vi "Initialize-object.vi"(8 "error in (no error)":errorcluster, 10 "Settings":T1, 11 "Base path":path) -> (0 "error out":errorcluster, 3 "Errors out":T3)   [LabVIEW 2013, in "CameraVision.lvlib" / "CV-Errors.lvclass"]
uses:
  CV-Errors.lvclass
  Object-reference.ctl
  Settings.ctl
  Languages.ctl
  CV-Errors.lvclass/CV-Errors.ctl
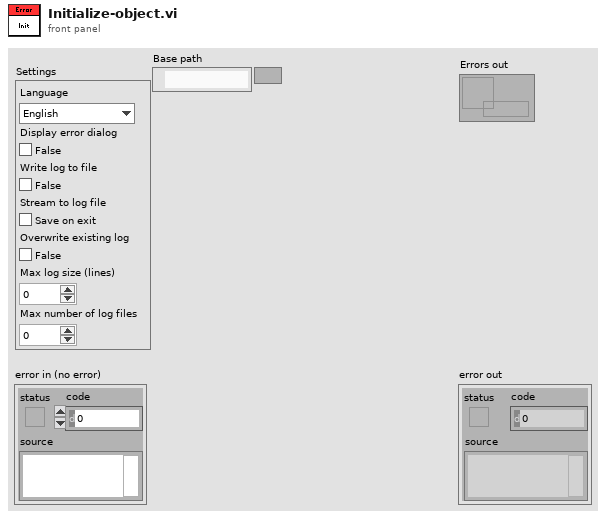
[diagram p1: front panel]
types:
  T1 = typedef "CameraVision.lvlib/CV-Errors.lvclass/Settings.ctl" = cluster{"Language":T2, "Display error dialog":bool, "Write log to file":bool, "Stream to log file":bool, "Overwrite existing log":bool, "Max log size":i32, "Max number of log files":i32}
  T2 = typedef "CameraVision.lvlib/CV-Errors.lvclass/Languages.ctl" = enum16{"English"}
  T3 = typedef "CameraVision.lvlib/CV-Errors.lvclass/Object-reference.ctl" = refnum<data-value>
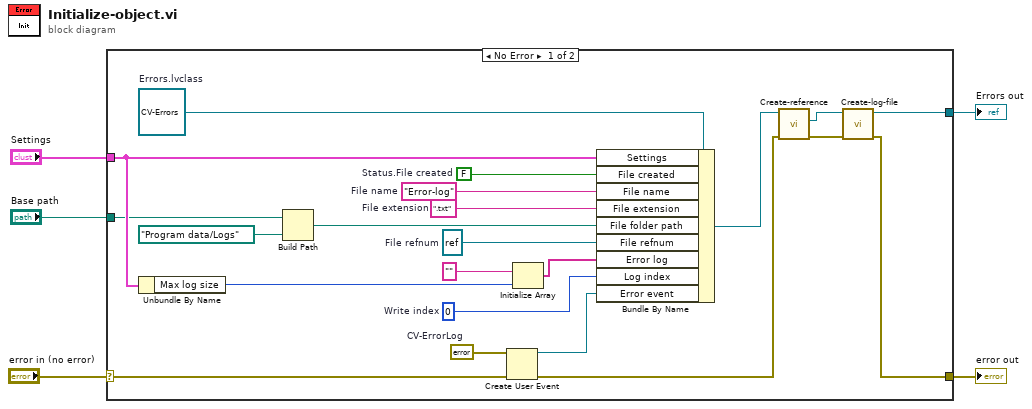
[diagram p0: block diagram]
diagram:
  n1 = case shown="No Error" "error in (no error)" {
    selector: "error in (no error)" -> [w9 w28]
    tunnel: [w17 w28] -> w4
    tunnel: [w16 _] -> w3
    tunnel: "Settings" -> [w13 _]
    tunnel: "Base path" -> [w7 _]
    frame No Error {
      w8 = errorcluster {"status"=FALSE, "code"=0, "source"=""}  # CV-ErrorLog
      w14 = FALSE  # Status.File created
      w15 = refnum<class "CV-Errors.lvclass"> refnum  # Errors.lvclass
      w21 = 0  # Write index
      w24 = refnum<file> refnum  # File refnum
      w26 = ".txt"  # File extension
      w27 = "Error-log"  # File name
      n2 = Unbundle By Name(w13) -> ("Max log size"=w12:i32)
      n3 = Build Path(base path=w7, name or relative path=path "Program data/Logs") -> (appended path=w25:path)
      n4 = Create User Event(user event datatype=w8, error in=w9) -> (user event=w10:refnum<user-event>, error out=w11:errorcluster)
      n5 = Initialize Array("", w12) -> (w23:string[])
      n6 = Bundle By Name(cluster=w15, "Settings"=w13, "File created"=w14, "File name"=w27, "File extension"=w26, "File folder path"=w25, "File refnum"=w24, "Error log"=w23, "Log index"=w21, "Error event"=w10) -> (w20:refnum<class "CV-Errors.lvclass">)
      n7 = call "Create-reference.vi"("error in (no error)"=w11, "Errors in"=w20) -> ("error out"=w18:errorcluster, "Errors reference"=w19:T3)  [unwired: 7 in, 1 out]
      n8 = call "Create-log-file.vi"("error in (no error)"=w18, "Errors in"=w19) -> ("error out"=w17:errorcluster, "Errors out"=w16:T3)  [unwired: 8 in]
    }
    frame Error {
    }
  }
  "error out" <- w4
  "Errors out" <- w3
